vi "Launch Debugger.vi"(8 "error in (no error)":errorcluster, 10 "Parent In":refnum<class "Module.lvclass">, 11 "Debug GUI Launcher in":refnum<class "Debug GUI Launcher.lvclass">) -> (0 "error out":errorcluster, 2 "Parent":refnum<class "Module.lvclass">)   [LabVIEW 2020, in "VolatusGUI.lvlib" / "Debug GUI Launcher.lvclass"]
uses:
  Debug GUI Launcher.lvclass
  Volatus/Module/Module.lvclass
  Debug GUI Module/Debug GUI Module.lvclass
  C:/dev/lv20CE/relink/lv-volatus/Volatus/Module/Module.lvclass
  VolatusConfig/VolatusConfigElement/VolatusConfigElement.lvclass
  Debug GUI Launcher.lvclass/Debug GUI Launcher.ctl
  C:/dev/lv20CE/relink/lv-volatus/VolatusGUI/Debug GUI Module/Debug GUI Module.lvclass
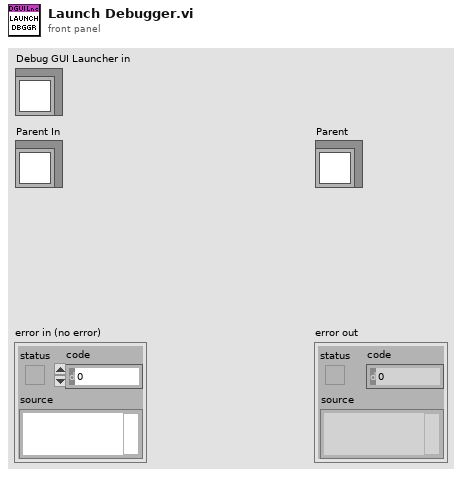
[diagram p1: front panel]
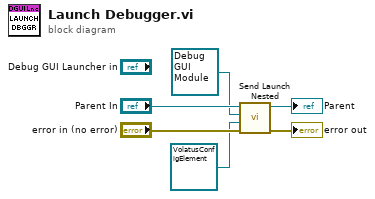
[diagram p0: block diagram]
diagram:
  n1 = call "Send Launch Nested.vi"("error in (no error)"="error in (no error)", "Config Element"=refnum<class "VolatusConfigElement.lvclass"> refnum, "Nested Module"=refnum<class "Debug GUI Module.lvclass"> refnum ("VolatusGUI:Debug GUI Module.lvclass"), "Module in"="Parent In") -> ("error out"=→"error out":errorcluster, "Module out"=→"Parent":refnum<class "Module.lvclass">)  [unwired: 6 in]
